vi "全局.vi"() -> ()   [LabVIEW 2011]
panel:
  in  "TestAction":enum16{"start", "stop", "pause", "reset"}(ring)
  out "Test Status":refnum<vi>
  in  "printpath":string
  in  "print templete":bool
  out "logsetting":dbl
  in  "manual stop":bool
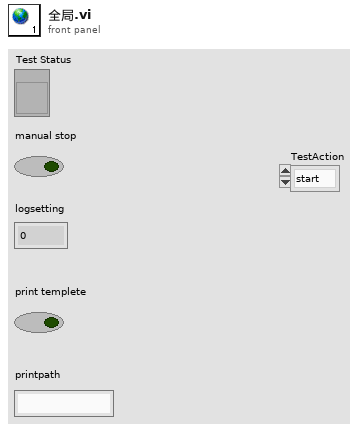
[diagram p1: front panel]
diagram:
